vi "receive_data.vi"(0 "存盘":bool, 5 "error in (no error)":errorcluster, 9 "file path (dialog if empty)":path=path "E:/测试数据/新芯片", 11 "Receive nums(70倍数)":i32) -> (4 "timeout?":bool, 6 "error out":errorcluster, 10 "VISA bytes now":i32)   [LabVIEW 2023, in "BT-Android_interface.lvlib"]
uses:
  BT-Android_interface.lvlib
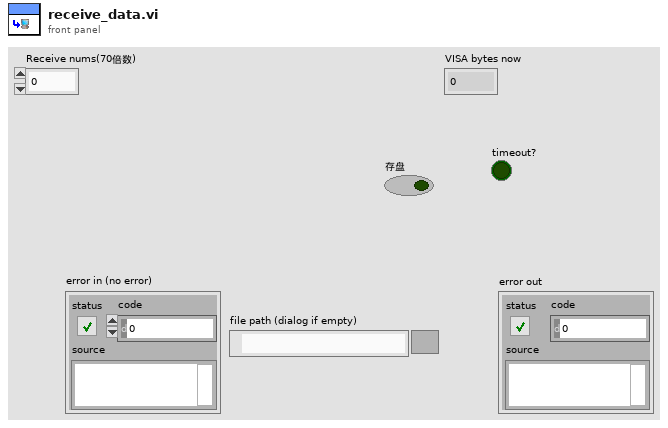
[diagram p1: front panel]
types:
  T1 = enum16{"init", "broadcast_data", "receive_data", "close", "clear_visa"}
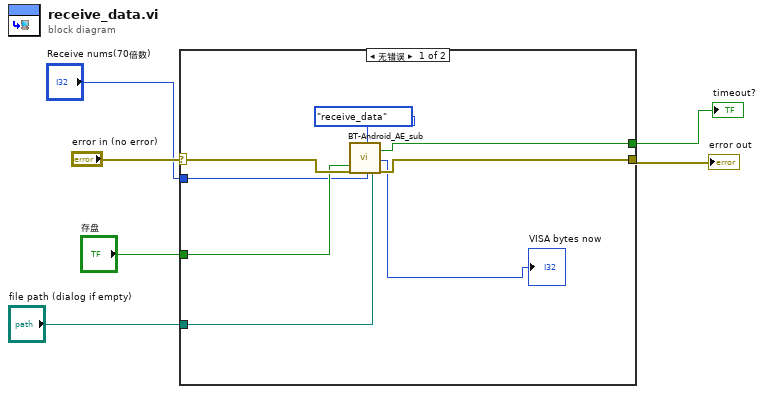
[diagram p0: block diagram]
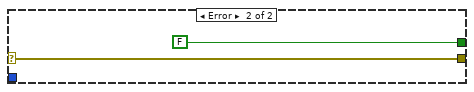
[diagram p2: hidden frame]
diagram:
  n1 = case shown="无错误" "error in (no error)" {
    selector: "error in (no error)" -> [w14 w16]
    tunnel: [w13 w16] -> w5
    tunnel: [w12 FALSE ("timeout?")] -> w4
    tunnel: "存盘" -> [w10 _]
    tunnel: "file path (dialog if empty)" -> [w9 _]
    tunnel: "Receive nums(70倍数)" -> [w8 _]
    frame No Error {
      n2 = call "BT-Android_AE_sub.vi"("存盘"=w10, "error in (no error)"=w14, "mode"=T1."receive_data", "Receive from Instr(bytes)\n(最好70倍数)"=w8, "file path (dialog if empty)"=w9) -> ("timeout?"=w12:bool, "VISA bytes now"=→"VISA bytes now":i32, "error IO"=w13:errorcluster)  [unwired: 12 in]
    }
    frame Error {
    }
  }
  "error out" <- w5
  "timeout?" <- w4
